vi "initialize.vi"(8 "error in (no error)":errorcluster, 11 "configuration []":T1[](array[typedef])) -> (0 "error out":errorcluster, 3 "runtime_data":variant)   [LabVIEW 2015, in "lv-calibration.lvlib"]
uses:
  lv-calibration.lvlib
  _controls/configuration.ctl
  _controls/type.ctl
  _controls/point.ctl
  _controls/error.ctl
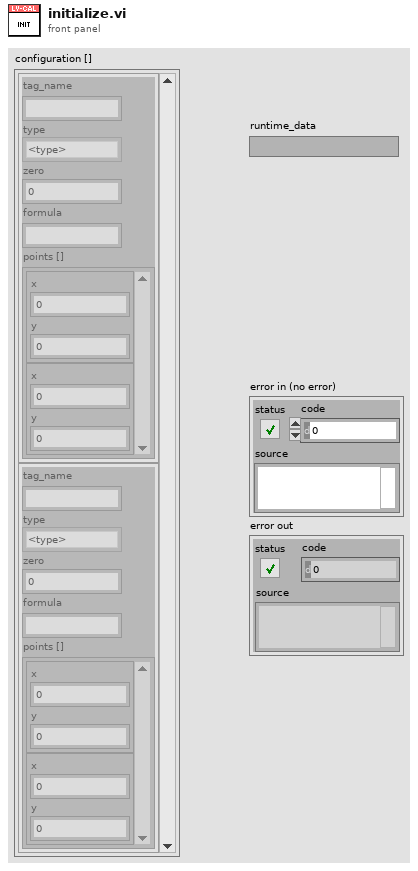
[diagram p1: front panel]
types:
  T1 = typedef "lv-calibration.lvlib/configuration.ctl" = cluster{"tag_name":string, "type":T2, "zero":dbl, "formula":string, "points []":T3[]}
  T2 = typedef "lv-calibration.lvlib/type.ctl" = enum16{"<type>", "slope_intercept", "linear_fit", "polynomial_fit", "interpolate", "formula"}
  T3 = typedef "lv-calibration.lvlib/point.ctl" = cluster{"x":dbl, "y":dbl}
  T4 = typedef "lv-calibration.lvlib/error.ctl" = enum16{"<error>", "unsupported_calibration_type", "tag_name_not_found", "duplicate_tag_names", "slope_intercept_bad_points", "formula_empty"}
  T5 = typedef "lv-calibration.lvlib/runtime.ctl" = cluster{"tag_name":string, "type":T2, "offset":dbl, "slope":dbl, "formula":string, "x []":dbl[], "y []":dbl[]}
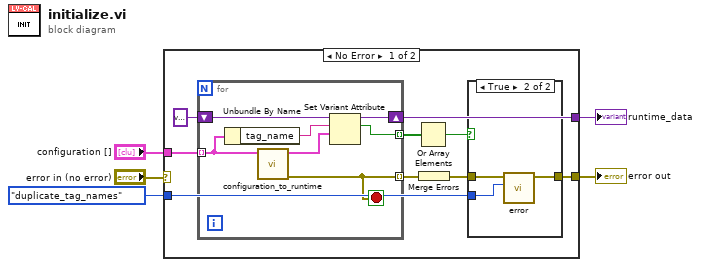
[diagram p0: block diagram]
diagram:
  n1 = case shown="No Error" "error in (no error)" {
    selector: "error in (no error)" -> [_ w26]
    tunnel: "configuration []" -> [w14 _]
    tunnel: [w12 _] -> w4
    tunnel: [w8 w26] -> w2
    tunnel: error."duplicate_tag_names" ("error") -> [w7 _]
    frame No Error {
      n2 = for {
        tunnel: w14 -> [w21] mode=indexing
        shift-right: [w24] -> w12
        shift-left: variant -> [w25]
        tunnel: [w22] -> w11 mode=indexing
        tunnel: [w19] -> w10 mode=indexing
        stop <- w19 stop-if-true
        n3 = Unbundle By Name(w21) -> ("tag_name"=w23:string)
        n4 = call "configuration_to_runtime.vi"("configuration"=w21) -> ("error out"=w19:errorcluster, "runtime"=w20:T5)  [unwired: 9 in]
        n5 = Set Variant Attribute(Variant=w25, name=w23, value=w20) -> (Variant out=w24:variant, replaced=w22:bool)  [unwired: 1 in, 1 out]
      }
      n6 = Or Array Elements(Boolean array=w11) -> (logical OR=w6:bool)
      n7 = Merge Errors(w10) -> (w9:errorcluster)
      n8 = case shown="True" w6 {
        tunnel: w9 -> [w15 w18]
        tunnel: [w15 w17] -> w8
        tunnel: w7 -> [_ w16]
        frame False {
        }
        frame True {
          n9 = call "error.vi"("error"=w16, "error in (no error)"=w18) -> ("error out"=w17:errorcluster)  [unwired: 9 in]
        }
      }
    }
    frame Error {
    }
  }
  "error out" <- w2
  "runtime_data" <- w4
